vi "password.vi"(9 "error in (no error)":errorcluster) -> (4 "done":bool, 6 "result":bool, 10 "This VI":refnum<vi>, 15 "error out":errorcluster)   [LabVIEW 2019]
panel:
  in  "Password":string
  in  "User Name":string
  out "String":string="Please insert User Name and Password"
  in  "Cancel":bool
  in  "OK2":bool
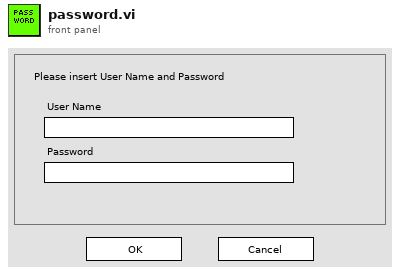
[diagram p1: front panel]
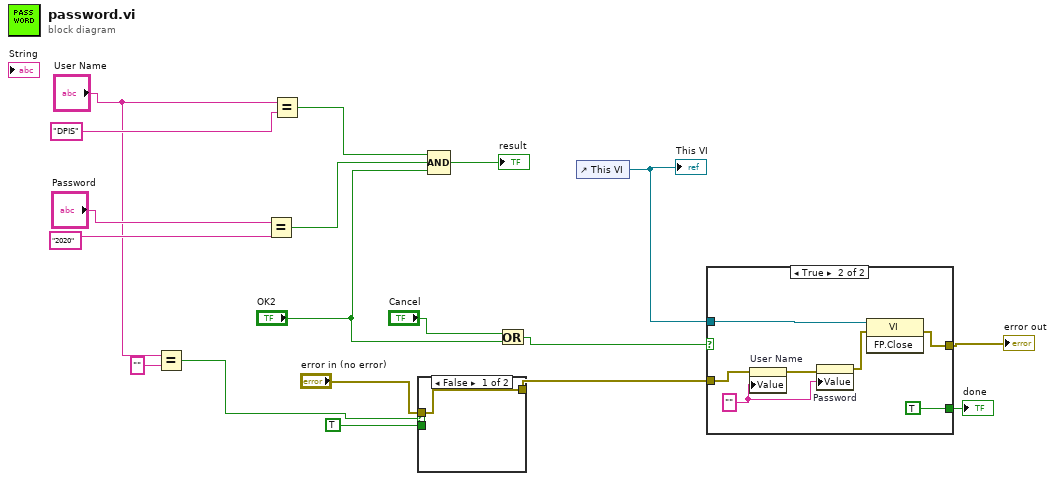
[diagram p0: block diagram]
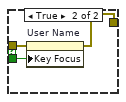
[diagram p2: hidden frame]
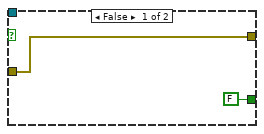
[diagram p3: hidden frame]
diagram:
  n1 = Equal?(x="User Name", y="") -> (x = y?=w2:bool)
  n2 = Equal?(x="Password", y="2020") -> (x = y?=w14:bool)
  n3 = Equal?(x="User Name", y="DPIS") -> (x = y?=w15:bool)
  n4 = case shown="False" w2 {
    tunnel: "error in (no error)" -> [w19 w22]
    tunnel: [w19 w21] -> w6
    tunnel: TRUE ("Key Focus") -> [_ w20]
    frame False {
    }
    frame True {
      n5 = property on="User Name" class="Str"(error in=w22, "Key Focus"=w20) -> (error out=w21:errorcluster)  [unwired: 1 in, 1 out]
    }
  }
  n6 = Compound Arithmetic op=AND(w15, w14, "OK2") -> (→"result":bool)
  n7 = Or(x="Cancel", y="OK2") -> (x .or. y?=w11:bool)
  n8 = control-ref of="This VI"() -> (w9:refnum<vi>)
  "This VI" <- w9
  n9 = case shown="True" w11 {
    tunnel: w9 -> [_ w31]
    tunnel: w6 -> [w24 w29]
    tunnel: [w24 w30] -> w8
    tunnel: [FALSE ("Key Focus") TRUE ("Key Focus")] -> w1
    frame False {
    }
    frame True {
      w26 = "" ("User Name")
      n10 = property on="User Name" class="Str"(error in=w29, "Value"=w26) -> (error out=w28:errorcluster)  [unwired: 1 in, 1 out]
      n11 = property on="Password" class="Str"(error in=w28, "Value"=w26) -> (error out=w27:errorcluster)  [unwired: 1 in, 1 out]
      n12 = invoke class="VI" method="FP.Close"(reference=w31, error in=w27) -> (error out=w30:errorcluster)  [unwired: 1 in, 2 out]
    }
  }
  "error out" <- w8
  "done" <- w1
